vi "AuMT8852B EDR Maximum Input Power Extended Results LEG.vi"(5 "Stage":T1(ring), 8 "error in (no error)":errorcluster, 11 "VISA session":refnum<visa-resource-name>) -> (0 "error out":errorcluster, 2 "error code":i32, 3 "VISA session out":refnum<visa-resource-name>, 4 "Results":T2 {"Overall BER" format="%.2e"; "Overall BER" format="%.2e"})   [LabVIEW 2017]
doc: "Anritsu MT8852B Bluetooth Tester\n\n<B>NOTE:</B> USE THIS VI ONLY FOR MT8852B FIRMWARE VERSIONS UP TO AND INCLUDING 4.08.100\n\nReturns the results of the EDR Maximum Input Power test.\n\nINPUTS\nStage - results of the individual hopping stages of the test.\n\nOUTPUTS\nResults - measurements made during the test."
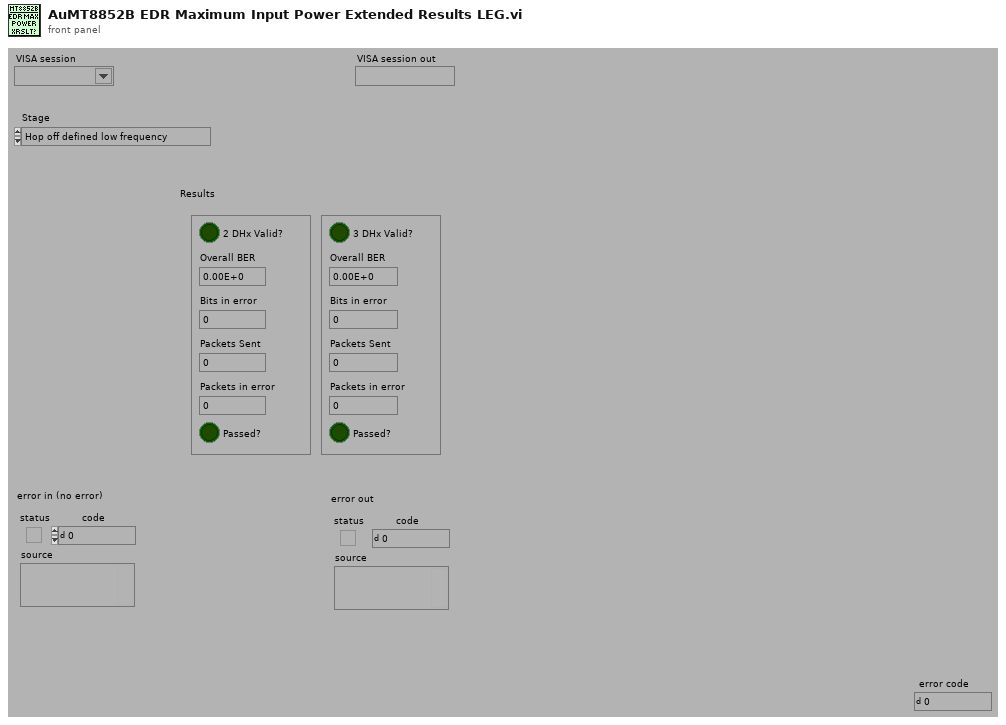
[diagram p1: front panel]
types:
  T1 = enum16{"Hop off defined low frequency", "Hop off defined medium frequency", "Hop off defined high frequency", "Hop on any channels"}
  T2 = cluster{"2 DHx Valid?":bool, "Overall BER":dbl, "Bits in error":u32, "Packets Sent":u32, "Passed?":bool, "Packets in error":u32, "3 DHx Valid?":bool, "Overall BER":dbl, "Bits in error":u32, "Packets Sent":u32, "Passed?":bool, "Packets in error":u32}
  T3 = enum16{"Simulate", "Range check", "Cache", "Query instrument status"}
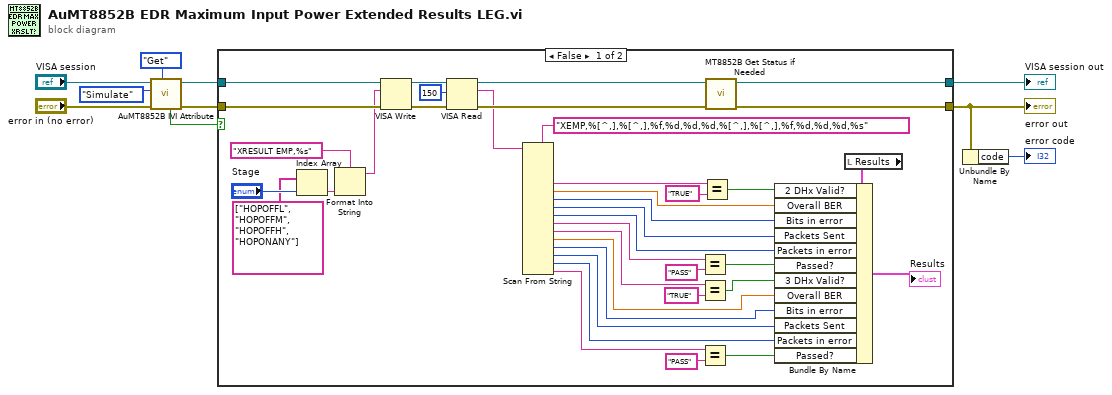
[diagram p0: block diagram]
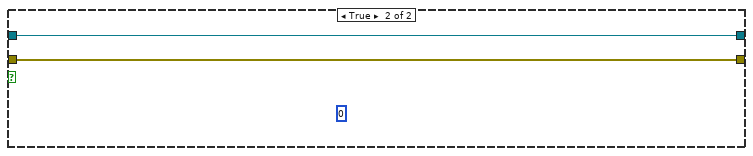
[diagram p2: hidden frame]
diagram:
  n1 = call <instrlib>:"AuMT8852B IVI Attribute.vi"("Set/Get (Set)"=enum16{"Set", "Get"}."Get", "error in (no error)"="error in (no error)", "Flag (Simulate)"=T3."Simulate", "VISA session"="VISA session") -> ("error out"=w7:errorcluster, "VISA session out"=w9:refnum<visa-resource-name>, "Value out"=w3:bool)  [unwired: 5 in]
  n2 = case shown="False" w3 {
    tunnel: [w42 w50] -> w10
    tunnel: [w41 w49] -> w1
    tunnel: w9 -> [w48 w50]
    tunnel: w7 -> [w47 w49]
    frame False {
      n3 = Index Array(array=string[] ["HOPOFFL", "HOPOFFM", "HOPOFFH", "HOPONANY"], index="Stage") -> (element=w28:string)
      n4 = Format Into String(format string="XRESULT EMP,%s" ("write buffer (\"\")"), w28) -> (resulting string=w25:string)  [unwired: 2 in, 1 out]
      n5 = VISA Write(VISA resource name=w48, write buffer=w25, error in (no error)=w47) -> (VISA resource name out=w46:refnum<visa-resource-name>, error out=w45:errorcluster)  [unwired: 1 out]
      n6 = VISA Read(VISA resource name=w46, byte count=u32 150 ("byte count (0)"), error in (no error)=w45) -> (VISA resource name out=w40:refnum<visa-resource-name>, read buffer=w23:string, error out=w39:errorcluster)  [unwired: 1 out]
      n7 = Scan From String(format string="XEMP,%[^,],%[^,],%f,%d,%d,%d,%[^,],%[^,],%f,%d,%d,%d,%s" ("Format String"), input string=w23) -> (output 2=w22:string, output 3=w21:dbl, output 4=w20:i32, output 5=w19:i32, output 6=w18:i32, output 7=w17:string, output 8=w16:string, output 9=w15:dbl, output 10=w14:i32, output 11=w13:i32, output 12=w12:i32, output 13=w11:string)  [unwired: 16 in, 3 out]
      n8 = Equal?(x=w17, y="PASS") -> (x = y?=w34:bool)
      n9 = Equal?(x=w16, y="TRUE") -> (x = y?=w32:bool)
      n10 = Equal?(x=w11, y="PASS") -> (x = y?=w31:bool)
      n11 = Equal?(x=w22, y="TRUE") -> (x = y?=w36:bool)
      n12 = call <instrlib>:"MT8852B Get Status if Needed.vi"("error in (no error)"=w39, "VISA session"=w40) -> ("error out"=w41:errorcluster, "VISA session out"=w42:refnum<visa-resource-name>)  [unwired: 8 in]
      n13 = local read "Results"() -> (w37:T2)
      n14 = Bundle By Name(cluster=w37, "2 DHx Valid?"=w36, "Overall BER"=w21, "Bits in error"=w20, "Packets Sent"=w19, "Packets in error"=w18, "Passed?"=w34, "3 DHx Valid?"=w32, "Overall BER"=w15, "Bits in error"=w14, "Packets Sent"=w13, "Packets in error"=w12, "Passed?"=w31) -> (→"Results":T2)
    }
    frame True {
      (unwired) u8 0
    }
  }
  "error out" <- w1
  "VISA session out" <- w10
  n15 = Unbundle By Name(w1) -> ("code"=→"error code":i32)
